vi "Three Button Dialog CORE-WithTimeout.vi"(0 "message":string, 1 "Window Title (\"\")":string, 3 "Justify Message (Left)":enum16{"Left", "Center", "Right"}(ring), 7 "Timeout(s)":i32=-1, 11 "error in (no error)":errorcluster, 12 "Keyboard Shortcuts (Left is <Enter>)":T1={"Left Button Key Shortcut"={"Control"=FALSE, "Shift"=FALSE, "Key"="<Enter>"}, "Center Button Key Shortcut"={"Control"=FALSE, "Shift"=FALSE, "Key"=""}, "Right Button Key Shortcut"={"Control"=FALSE, "Shift"=FALSE, "Key"=""}}, 13 "Enable(t)":bool=TRUE, 14 "Allow user to close window? (TRUE)":bool=TRUE) -> (2 "OK(?)":bool, 4 "Which Button?":T2(ring)=enum."Center Button", 15 "error out":errorcluster)   [LabVIEW 2018]
doc: "Displays text in a dialog with three buttons. The output enum indicates which of the three buttons the user chose, or it indicates that the user closed the dialog without making any choice."
uses:
  <vilib>/Utility/miscctls.llb/LVRectTypeDef.ctl
panel:
  in  "OK":string="OK"
  out "C-Message":string
  in  "Right Button":bool
  in  "Center Button":bool
  in  "Left Button":bool
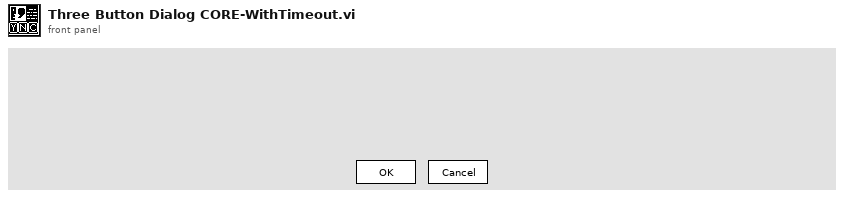
[diagram p1: front panel]
types:
  T1 = cluster{"Left Button Key Shortcut":cluster{"Control":bool, "Shift":bool, "Key":string}, "Center Button Key Shortcut":cluster{"Control":bool, "Shift":bool, "Key":string}, "Right Button Key Shortcut":cluster{"Control":bool, "Shift":bool, "Key":string}}
  T2 = enum16{"Left Button", "Center Button", "Right Button", "Window Close"}
  T3 = cluster{"left":i16, "top":i16, "right":i16, "bottom":i16}
  T4 = cluster{"Control":bool, "Shift":bool, "Key":string}
  T5 = cluster{bool, "Control":bool, "Shift":bool, "Key":string}
  T6 = typedef "LVRectTypeDef.ctl" = cluster{"Left":i16, "Top":i16, "Right":i16, "Bottom":i16}
  T7 = typedef "LVBoundsTypeDef.ctl" = cluster{"Width":u32, "Height":u32}
  T8 = typedef "LVPointTypeDef.ctl" = cluster{"Horizontal":i16, "Vertical":i16}
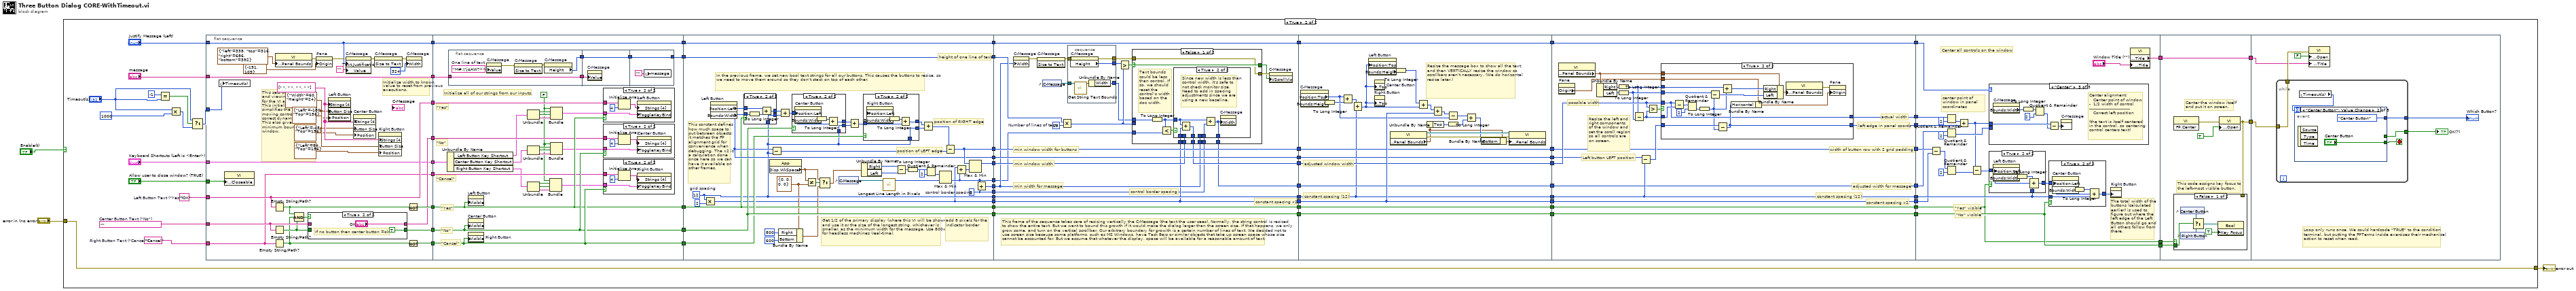
[diagram p0: block diagram]
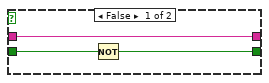
[diagram p3: hidden frame]
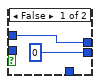
[diagram p7: hidden frame]
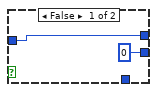
[diagram p8: hidden frame]
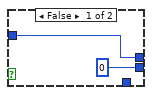
[diagram p9: hidden frame]
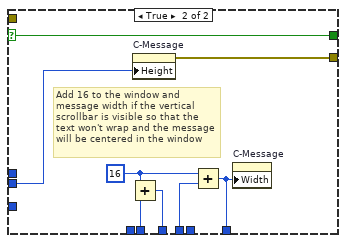
[diagram p11: hidden frame]
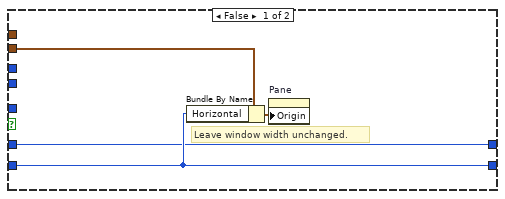
[diagram p12: hidden frame]
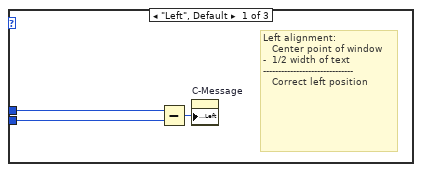
[diagram p13: hidden frame]
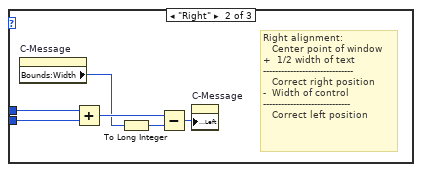
[diagram p14: hidden frame]
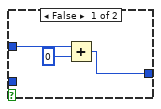
[diagram p15: hidden frame]
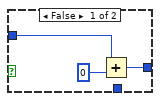
[diagram p16: hidden frame]
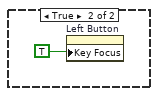
[diagram p17: hidden frame]
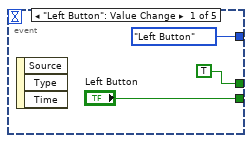
[diagram p18: hidden frame]
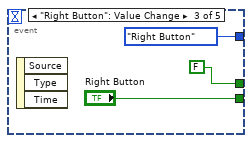
[diagram p19: hidden frame]
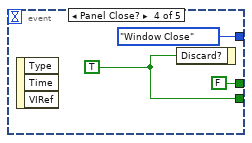
[diagram p20: hidden frame]
diagram:
  n1 = case shown="True" "Enable(t)" {
    tunnel: "error in (no error)" -> [_ w9]
    tunnel: [_ w9] -> w1
    frame False {
    }
    frame True {
      w15 = "Cancel"  # Right Button Text ("Cancel")
      w16 = ""  # Center Button Text ("No")
      w17 = "OK"  # Left Button Text ("Yes")
      n2 = Equal?(x=-1, y="Timeout(s)") -> (x = y?=w5:bool)
      n3 = Multiply(x="Timeout(s)", y=1000) -> (x*y=w8:i32)
      n4 = Select(t="Timeout(s)", s=w5, f=w8) -> (s? t:f=w4:i32)
      n5 = flat-sequence {
        tunnel: [w94] -> w75
        tunnel: [w96] -> w74
        tunnel: [w95] -> w73
        tunnel: [w90] -> w72
        tunnel: [w91] -> w71
        tunnel: [w88] -> w70
        tunnel: [w87] -> w69
        tunnel: w17 -> [w90]
        tunnel: w16 -> [w89]
        tunnel: w15 -> [w88]
        tunnel: "Justify Message (Left)" -> [w87]
        tunnel: "Keyboard Shortcuts (Left is <Enter>)" -> [w84]
        tunnel: [w84] -> w68
        tunnel: "message" -> [w83]
        tunnel: [w83] -> w67
        tunnel: "Allow user to close window? (TRUE)" -> [w82]
        tunnel: w4 -> [w76]
        tunnel: w75 -> [w138]
        tunnel: [w138] -> w66
        tunnel: w74 -> [w137]
        tunnel: [w137] -> w65
        tunnel: w73 -> [w136]
        tunnel: [w136] -> w64
        tunnel: w72 -> [w135]
        tunnel: w71 -> [w134]
        tunnel: w70 -> [w133]
        tunnel: w69 -> [w132]
        tunnel: [w132] -> w63
        tunnel: [w128] -> w62
        tunnel: w68 -> [w131]
        tunnel: w67 -> [w127]
        tunnel: [w199] -> w61
        tunnel: [w196] -> w60
        tunnel: [w195] -> w59
        tunnel: [w178] -> w58
        tunnel: [w160] -> w57
        tunnel: w66 -> [w188]
        tunnel: w65 -> [w190]
        tunnel: [w190] -> w56
        tunnel: w64 -> [w186]
        tunnel: [w186] -> w55
        tunnel: [w171] -> w54
        tunnel: w63 -> [w181]
        tunnel: [w181] -> w53
        tunnel: w62 -> [w180]
        tunnel: [w180] -> w52
        tunnel: [w169] -> w51
        tunnel: [w168] -> w50
        tunnel: w61 -> [w234]
        tunnel: [w233] -> w49
        tunnel: w60 -> [w240]
        tunnel: [w240] -> w48
        tunnel: w59 -> [w239]
        tunnel: [w239] -> w47
        tunnel: w58 -> [w238]
        tunnel: [w238] -> w46
        tunnel: w57 -> [w227]
        tunnel: [w227] -> w45
        tunnel: w56 -> [w237]
        tunnel: [w237] -> w44
        tunnel: w55 -> [w236]
        tunnel: [w236] -> w43
        tunnel: w54 -> [w228]
        tunnel: [w232] -> w42
        tunnel: w53 -> [w235]
        tunnel: [w235] -> w41
        tunnel: w52 -> [w230]
        tunnel: w51 -> [w226]
        tunnel: w50 -> [w225]
        tunnel: w49 -> [w289]
        tunnel: [w289] -> w40
        tunnel: w48 -> [w288]
        tunnel: [w288] -> w39
        tunnel: w47 -> [w287]
        tunnel: [w287] -> w38
        tunnel: w46 -> [w280]
        tunnel: [w280] -> w37
        tunnel: w45 -> [w297]
        tunnel: [w297] -> w36
        tunnel: w44 -> [w286]
        tunnel: [w286] -> w35
        tunnel: w43 -> [w285]
        tunnel: [w285] -> w34
        tunnel: w42 -> [w284]
        tunnel: [w284] -> w33
        tunnel: w41 -> [w283]
        tunnel: [w283] -> w32
        tunnel: w40 -> [w324]
        tunnel: [w319] -> w31
        tunnel: w39 -> [w312]
        tunnel: [w312] -> w30
        tunnel: w38 -> [w318]
        tunnel: w37 -> [w317]
        tunnel: [w317] -> w29
        tunnel: w36 -> [w311]
        tunnel: [w311] -> w28
        tunnel: [w315] -> w27
        tunnel: w35 -> [w310]
        tunnel: [w310] -> w26
        tunnel: w34 -> [w309]
        tunnel: [w309] -> w25
        tunnel: w33 -> [w306]
        tunnel: [w306] -> w24
        tunnel: w32 -> [w308]
        tunnel: [w308] -> w23
        tunnel: [w349] -> w22
        tunnel: w31 -> [w368]
        tunnel: w30 -> [w361]
        tunnel: w29 -> [w365]
        tunnel: w28 -> [w360]
        tunnel: w27 -> [w367]
        tunnel: w26 -> [w348]
        tunnel: w25 -> [w347]
        tunnel: w24 -> [w353]
        tunnel: w23 -> [w354]
        tunnel: [w348] -> w21
        tunnel: [w347] -> w20
        tunnel: w22 -> [w404]
        tunnel: w21 -> [w400]
        tunnel: w20 -> [w401]
        tunnel: [w402] -> w19
        tunnel: [w404] -> w18
        tunnel: w19 -> [w412]
        tunnel: w18 -> [w413]
        frame #0 {
          w104 = string[] [" ", " ", " ", " "] ("Strings [4]")
          w103 = cluster{"Width":u32, "Height":u32} {"Width"=60, "Height"=24} ("Button Size")
          # "Initialize width to known value to reset from previous executions."
          # "This sets up initial sizes and viewing rectangles\nfor the VI and its controls. This initialization\nsimplifies the task of moving controls to their\ncorrect dynamic locations. This also gives us our\nminimum bounds for the window."
          n6 = local write "Timeout(s)"(w76) -> ()
          n7 = property class="VI"("Front Panel Window:Closeable"=w82) -> ()  [unwired: 2 in, 2 out]
          n8 = Empty String/Path?(string/path=w90) -> (empty?=w98:bool)
          n9 = Empty String/Path?(string/path=w89) -> (empty?=w86:bool)
          n10 = Empty String/Path?(string/path=w88) -> (empty?=w85:bool)
          n11 = property class="VI"("Front Panel Window:Panel Bounds"=T3 {"left"=338, "top"=316, "right"=686, "bottom"=392} ("Front Panel.PanelBounds")) -> (error out=w81:errorcluster)  [unwired: 2 in, 1 out]
          n12 = Compound Arithmetic op=AND(w98, w85, w86) -> (w97:bool)
          n13 = case shown="True" w97 {
            tunnel: w86 -> [w107 _]
            tunnel: [w106 TRUE] -> w96
            tunnel: w89 -> [w105 _]
            tunnel: [w105 "OK"] -> w91
            frame False {
              n14 = Not(x=w107) -> (.not. x?=w106:bool)
            }
            frame True {
              # "If no button then center button =ok"
            }
          }
          n15 = property on="Pane" class="Pane"(error in=w81, "Origin"=cluster{"Horizontal":i16, "Vertical":i16} {"Horizontal"=-191, "Vertical"=109} ("Front Panel.Origin")) -> (error out=w80:errorcluster)  [unwired: 1 in, 1 out]
          n16 = property on="Left Button" class="Bool"("Strings [4]"=w104, "Button Size"=w103, "Position"=cluster{"Left":i32, "Top":i32} {"Left"=-180, "Top"=156}) -> ()  [unwired: 2 in, 2 out]
          n17 = property on="C-Message" class="Str"(error in=w80, "Text.Justification"=w87, "Value"="") -> (error out=w99:errorcluster)  [unwired: 1 in, 1 out]
          n18 = property on="Center Button" class="Bool"("Strings [4]"=w104, "Button Size"=w103, "Position"=cluster{"Left":i32, "Top":i32} {"Left"=-48, "Top"=156}) -> ()  [unwired: 2 in, 2 out]
          n19 = invoke on="C-Message" class="Str" method="Size to Text"(error in=w99) -> (error out=w78:errorcluster)  [unwired: 2 in, 2 out]
          n20 = property on="Right Button" class="Bool"("Strings [4]"=w104, "Button Size"=w103, "Position"=cluster{"Left":i32, "Top":i32} {"Left"=84, "Top"=156}) -> ()  [unwired: 2 in, 2 out]
          n21 = property on="C-Message" class="Str"(error in=w78, "Width"=u32 324 ("Size:Width")) -> ()  [unwired: 1 in, 2 out]
          n22 = Not(x=w98) -> (.not. x?=w95:bool)
          n23 = Not(x=w85) -> (.not. x?=w94:bool)
        }
        frame #1 {
          w112 = FALSE
          # "\"Cancel\""
          # "\"No\""
          # "\"Yes\""
          # "\"Cancel\""
          # "\"No\""
          # "\"Yes\""
          # "Initialize all of our strings from our inputs."
          n24 = Unbundle By Name(w131) -> ("Left Button Key Shortcut"=w125:T4, "Center Button Key Shortcut"=w117:T4, "Right Button Key Shortcut"=w111:T4)
          n25 = flat-sequence {
            tunnel: [w140] -> w130
            tunnel: w127 -> [w139]
            tunnel: [w139] -> w126
            tunnel: w130 -> [w145]
            tunnel: [w145] -> w129
            tunnel: w126 -> [w144]
            tunnel: w129 -> [w146]
            tunnel: [w146] -> w128
            frame #0 {
              w143 = "M#,\"jqAW?><"  # One line of text
              n26 = property on="C-Message" class="Str"("Value"=w143) -> (error out=w141:errorcluster)  [unwired: 2 in, 1 out]
              n27 = invoke on="C-Message" class="Str" method="Size to Text"(error in=w141) -> (error out=w142:errorcluster)  [unwired: 2 in, 2 out]
              n28 = property on="C-Message" class="Str"(error in=w142) -> ("Height"=w140:u32)  [unwired: 1 in, 2 out]
            }
            frame #1 {
              n29 = property on="C-Message" class="Str"("Value"=w144) -> ()  [unwired: 2 in, 2 out]
            }
            frame #2 {
              n30 = local write "message"("") -> ()
            }
          }
          n31 = property on="Left Button" class="Bool"("Visible"=w136) -> ()  [unwired: 2 in, 2 out]
          n32 = property on="Center Button" class="Bool"("Visible"=w137) -> ()  [unwired: 2 in, 2 out]
          n33 = property on="Right Button" class="Bool"("Visible"=w138) -> ()  [unwired: 2 in, 2 out]
          n34 = Unbundle(w125) -> ("Control"=w124:bool, "Shift"=w123:bool, "Key"=w122:string)
          n35 = Unbundle(w117) -> ("Control"=w120:bool, "Shift"=w119:bool, "Key"=w118:string)
          n36 = Unbundle(w111) -> ("Control"=w115:bool, "Shift"=w114:bool, "Key"=w113:string)
          n37 = Bundle(w112, "Control"=w115, "Shift"=w114, "Key"=w113) -> (w110:T5)  [unwired: 1 in]
          n38 = Bundle(w112, "Control"=w124, "Shift"=w123, "Key"=w122) -> (w121:T5)  [unwired: 1 in]
          n39 = Bundle(w112, "Control"=w120, "Shift"=w119, "Key"=w118) -> (w116:T5)  [unwired: 1 in]
          n40 = case shown="True" w136 {
            tunnel: w135 -> [_ w157]
            tunnel: w121 -> [_ w156]
            frame False {
            }
            frame True {
              n41 = Initialize Array(w157, 4 ("dimension size")) -> (w159:string[])
              n42 = property on="Left Button" class="Bool"("Strings [4]"=w159, "ToggleKeyBind"=w156) -> ()  [unwired: 2 in, 2 out]
            }
          }
          n43 = case shown="True" w137 {
            tunnel: w116 -> [_ w153]
            tunnel: w134 -> [_ w152]
            frame False {
            }
            frame True {
              n44 = Initialize Array(w152, 4 ("dimension size")) -> (w155:string[])
              n45 = property on="Center Button" class="Bool"("Strings [4]"=w155, "ToggleKeyBind"=w153) -> ()  [unwired: 2 in, 2 out]
            }
          }
          n46 = case shown="True" w138 {
            tunnel: w110 -> [_ w149]
            tunnel: w133 -> [_ w148]
            frame False {
            }
            frame True {
              n47 = Initialize Array(w148, 4 ("dimension size")) -> (w151:string[])
              n48 = property on="Right Button" class="Bool"("Strings [4]"=w151, "ToggleKeyBind"=w149) -> ()  [unwired: 2 in, 2 out]
            }
          }
        }
        frame #2 {
          w165 = T6 {"Left"=0, "Top"=0, "Right"=0, "Bottom"=0} ("Display:Primary Workspace")
          w169 = 8  # control border spacing
          w178 = 12  # grid spacing
          # "position of RIGHT edge"
          # "height of one line of text"
          # "add 8 pixels for the indicator border"
          # "Get 1/2 of the primary display (where this VI will be shown) and use it or the size of the longest string, whichever is smaller, as the minimum width for the message. Use 800x600 for headless machines (real-time)."
          # "This constant defines how much space to put between objects; it matches the FP alignment grid for convenience when debugging. The x2 is a calculation done once here so we can have it available on other frames."
          # "In the previous frame, we set new bool text strings for all our buttons. This causes the buttons to resize, so we need to move them around so they don't stack on top of each other."
          # "position of LEFT edge"
          n49 = Multiply(x=w178, y=2) -> (x*y=w160:i32)
          n50 = property on="Left Button" class="Bool"() -> ("Position:Left"=w195:i32, "Bounds:Width"=w192:u32)  [unwired: 2 in, 2 out]
          n51 = case shown="True" w186 {
            tunnel: w195 -> [w202 w207]
            tunnel: w192 -> [_ w206]
            tunnel: [w202 w205] -> w187
            tunnel: w178 -> [_ w203]
            tunnel: [0 w203] -> w185
            frame False {
            }
            frame True {
              n52 = To Long Integer(number=w206) -> (32bit integer=w204:i32)
              n53 = Add(x=w207, y=w204) -> (x+y=w205:i32)
            }
          }
          n54 = property class="App"() -> ("Disp.WkSpace"=w166:T6)  [unwired: 2 in, 2 out]
          n55 = Subtract(x=w195, y=w178) -> (x-y=w197:i32)
          n56 = Bundle By Name(cluster=w165, "Right"=i16 800, "Bottom"=i16 600) -> (w162:T6)
          n57 = Add(x=w187, y=w185) -> (x+y=w193:i32)
          n58 = case shown="True" w190 {
            tunnel: w193 -> [w216 w221]
            tunnel: [w216 w220] -> w191
            tunnel: [0 w217] -> w184
            tunnel: w178 -> [_ w217]
            frame False {
            }
            frame True {
              n59 = property on="Center Button" class="Bool"("Position:Left"=w221) -> ("Bounds:Width"=w219:u32)  [unwired: 2 in, 2 out]
              n60 = To Long Integer(number=w219) -> (32bit integer=w218:i32)
              n61 = Add(x=w218, y=w221) -> (x+y=w220:i32)
            }
          }
          n62 = Not Equal?(x=w166, y=w165) -> (x != y?=w167:bool)
          n63 = Select(t=w166, s=w167, f=w162) -> (s? t:f=w161:T6)
          n64 = control-ref of="C-Message"() -> (w182:refnum<vi>)
          n65 = Add(x=w191, y=w184) -> (x+y=w194:i32)
          n66 = Unbundle By Name(w161) -> ("Right"=w174:i16, "Left"=w173:i16)
          n67 = case shown="True" w188 {
            tunnel: w194 -> [w209 w214]
            tunnel: [w209 w210] -> w189
            tunnel: [0 w211] -> w183
            tunnel: w178 -> [_ w211]
            frame False {
            }
            frame True {
              n68 = property on="Right Button" class="Bool"("Position:Left"=w214) -> ("Bounds:Width"=w213:u32)  [unwired: 2 in, 2 out]
              n69 = To Long Integer(number=w213) -> (32bit integer=w212:i32)
              n70 = Add(x=w212, y=w214) -> (x+y=w210:i32)
            }
          }
          n71 = call <vilib>:"Longest Line Length in Pixels.vi"("String"=w182) -> ("longest line length"=w175:i32)  [unwired: 9 in]
          n72 = Subtract(x=w174, y=w173) -> (x-y=w177:i16)
          n73 = To Long Integer(number=w177) -> (32bit integer=w172:i32)
          n74 = Add(x=w189, y=w183) -> (x+y=w198:i32)
          n75 = Quotient & Remainder(x=w172, y=2) -> (floor(x/y)=w170:i32)  [unwired: 1 out]
          n76 = Max & Min(x=w170, y=w175) -> (min(x,y)=w168:i32)  [unwired: 1 out]
          n77 = Subtract(x=w198, y=w197) -> (x-y=w196:i32)
          n78 = Add(x=w160, y=w168) -> (x+y=w200:i32)
          n79 = Max & Min(x=w196, y=w200) -> (max(x,y)=w199:i32)  [unwired: 1 out]
          n80 = Add(x=w168, y=w169) -> (x+y=w171:i32)
        }
        frame #3 {
          w242 = u32 25  # Number of lines of text
          # "control border spacing"
          # "constant spacing x2"
          # "min window width for buttons"
          # "min window width"
          # "min width for message"
          # "This frame of the sequence takes care of resizing vertically the C-Message (the text the user sees). Normally, the string control is resized to show the entire text. But we want to bound this growth if it would make the dialog larger than the screen size. If that happens, we only grow some, and turn on the vertical scrollbar. Our arbitrary boundary for growith is a certain number of lines of text. We decided not to use screen size because some platforms, such as MS Windows, have Task Bars or similar objects that take up screen space whose size cannot be accounted for. But we assume that whatever the display, space will be available for a reasonable amount of text."
          n81 = property on="C-Message" class="Str"("Width"=w228) -> (error out=w231:errorcluster)  [unwired: 2 in, 1 out]
          n82 = invoke on="C-Message" class="Str" method="Size to Text"(error in=w231) -> (error out=w246:errorcluster)  [unwired: 2 in, 2 out]
          n83 = control-ref of="C-Message"() -> (w223:refnum<vi>)
          n84 = Multiply(x=w230, y=w242) -> (x*y=w241:u32)
          n85 = stacked-sequence {
            tunnel: w246 -> [w252]
            tunnel: [w251] -> w229
            tunnel: [w250] -> w224
            tunnel: w223 -> [w249]
            tunnel: [w247] -> w222
            frame #0 {
              n86 = property on="C-Message" class="Str"(error in=w252) -> (error out=w250:errorcluster, "Height"=w251:u32)  [unwired: 1 in, 1 out]
              n87 = call <vilib>:"Get String Text Bounds.vi"("String"=w249) -> ("Text bounds"=w248:T7)  [unwired: 10 in]
              n88 = Unbundle By Name(w248) -> ("Width"=w247:u32)
            }
          }
          n89 = Greater?(x=w229, y=w241) -> (0:w245:bool)
          n90 = case shown="False" w245 {
            selector: w245 -> [w264 w278]
            tunnel: [w263 w279] -> w244
            tunnel: [w264 w278] -> w243
            tunnel: w224 -> [w263 _]
            tunnel: w241 -> [_ w277]
            tunnel: [w257 w275] -> w233
            tunnel: w234 -> [w259 w276]
            tunnel: [w256 w272] -> w232
            tunnel: w228 -> [w258 w274]
            tunnel: w222 -> [w261 _]
            tunnel: w225 -> [w260 _]
            tunnel: w227 -> [w255 _]
            tunnel: w226 -> [w254 _]
            frame False {
              # "Text bounds could be less than control. If so, we should reset the control's width based on the doc width."
              n91 = To Long Integer(number=w261) -> (32bit integer=w253:i32)
              n92 = Less?(x=w253, y=w260) -> (x < y?=w262:bool)
              n93 = case shown="True" w262 {
                tunnel: w253 -> [_ w270]
                tunnel: w259 -> [w266 _]
                tunnel: w258 -> [w265 _]
                tunnel: [w266 w269] -> w257
                tunnel: [w265 w268] -> w256
                tunnel: w255 -> [_ w271]
                tunnel: w254 -> [_ w267]
                frame False {
                }
                frame True {
                  # "Since new width is less than control width, it's safe to not check monitor size. \nNeed to add in spacing adjustments since we are using a new baseline."
                  n94 = Add(x=w270, y=w271) -> (x+y=w269:i32)
                  n95 = Add(x=w270, y=w267) -> (x+y=w268:i32)
                  n96 = property on="C-Message" class="Str"("Width"=w268) -> ()  [unwired: 2 in, 2 out]
                }
              }
            }
            frame True {
              w273 = 16 ("x")
              # "Add 16 to the window and message width if the vertical scrollbar is visible so that the text won't wrap and the message will be centered in the window"
              n97 = Add(x=w273, y=w276) -> (x+y=w275:i32)
              n98 = property on="C-Message" class="Str"("Height"=w277) -> (error out=w279:errorcluster)  [unwired: 2 in, 1 out]
              n99 = Add(x=w273, y=w274) -> (x+y=w272:i32)
              n100 = property on="C-Message" class="Str"("Width"=w272) -> ()  [unwired: 2 in, 2 out]
            }
          }
          n101 = property on="C-Message" class="Str"(error in=w244, "VScrollVis"=w243) -> ()  [unwired: 1 in, 2 out]
        }
        frame #4 {
          # "adjusted window width"
          # "constant spacing (12)"
          # "Resize the message box to show all the text, and then VERTICALLY resize the window so scrollbars aren't necessary. (We do horizontal resize later.)"
          n102 = property on="C-Message" class="Str"() -> ("Position:Top"=w291:i32, "Bounds:Height"=w290:u32)  [unwired: 2 in, 2 out]
          n103 = To Long Integer(number=w290) -> (32bit integer=w296:i32)
          n104 = Add(x=w291, y=w296) -> (x+y=w281:i32)
          n105 = Add(x=w281, y=w280) -> (x+y=w282:i32)
          n106 = property on="Left Button" class="Bool"("Position:Top"=w282) -> ("Bounds:Height"=w293:u32)  [unwired: 2 in, 2 out]
          n107 = property on="Center Button" class="Bool"("Position:Top"=w282) -> ()  [unwired: 2 in, 2 out]
          n108 = property on="Right Button" class="Bool"("Position:Top"=w282) -> ()  [unwired: 2 in, 2 out]
          n109 = property class="VI"() -> (reference out=w303:refnum<vi>, error out=w304:errorcluster, "Front Panel Window:Panel Bounds"=w294:T6)  [unwired: 2 in]
          n110 = To Long Integer(number=w293) -> (32bit integer=w292:i32)
          n111 = Add(x=w292, y=w282) -> (x+y=w298:i32)
          n112 = Unbundle By Name(w294) -> ("Top"=w301:i16)
          n113 = Add(x=w298, y=w297) -> (x+y=w299:i32)
          n114 = Subtract(x=w299, y=w291) -> (x-y=w302:i32)
          n115 = To Long Integer(number=w301) -> (32bit integer=w295:i32)
          n116 = Add(x=w302, y=w295) -> (x+y=w300:i32)
          n117 = Bundle By Name(cluster=w294, "Bottom"=w300) -> (w305:T6)
          n118 = property class="VI"(reference=w303, error in=w304, "Front Panel Window:Panel Bounds"=w305) -> ()  [unwired: 2 out]
        }
        frame #5 {
          # "adjusted width for message"
          # "constant spacing x2"
          # "constant spacing (12)"
          # "Left button LEFT position"
          # "left edge in panel coords"
          # "width of button row with 2 grid padding"
          # "Resize the left and\nright components\nof the window and\nset the scroll region\nso all controls are \non screen."
          # "actual width"
          # "possible width"
          n119 = property class="VI"() -> ("Front Panel Window:Panel Bounds"=w321:T6)  [unwired: 2 in, 2 out]
          n120 = property on="Pane" class="Pane"() -> ("Origin"=w307:T8)  [unwired: 2 in, 2 out]
          n121 = Unbundle By Name(w321) -> ("Right"=w323:i16, "Left"=w322:i16)
          n122 = To Long Integer(number=w323) -> (32bit integer=w313:i32)
          n123 = To Long Integer(number=w322) -> (32bit integer=w314:i32)
          n124 = Subtract(x=w313, y=w314) -> (x-y=w325:i32)
          n125 = Subtract(x=w318, y=w317) -> (x-y=w316:i32)
          n126 = Greater?(x=w324, y=w325) -> (0:w320:bool)
          n127 = case shown="True" w320 {
            tunnel: w325 -> [w327 w346]
            tunnel: w324 -> [_ w333]
            tunnel: w313 -> [_ w341]
            tunnel: w314 -> [_ w342]
            tunnel: w321 -> [_ w343]
            tunnel: [w329 w335] -> w319
            tunnel: w307 -> [w328 w336]
            tunnel: w316 -> [w329 w334]
            tunnel: [w327 w333] -> w315
            frame False {
              # "Leave window width unchanged."
              n128 = Bundle By Name(cluster=w328, "Horizontal"=w329) -> (w326:T8)
              n129 = property on="Pane" class="Pane"("Origin"=w326) -> ()  [unwired: 2 in, 2 out]
            }
            frame True {
              n130 = Subtract(x=w333, y=w346) -> (x-y=w345:i32)
              n131 = Quotient & Remainder(x=w345, y=2) -> (floor(x/y)=w338:i32)  [unwired: 1 out]
              n132 = To Long Integer(number=w338) -> (32bit integer=w332:i32)
              n133 = Subtract(x=w342, y=w332) -> (x-y=w339:i32)
              n134 = Subtract(x=w334, y=w332) -> (x-y=w335:i32)
              n135 = Add(x=w341, y=w332) -> (x+y=w340:i32)
              n136 = Bundle By Name(cluster=w336, "Horizontal"=w335) -> (w330:T8)
              n137 = Bundle By Name(cluster=w343, "Right"=w340, "Left"=w339) -> (w337:T6)
              n138 = property class="VI"("Front Panel Window:Panel Bounds"=w337) -> (error out=w331:errorcluster)  [unwired: 2 in, 1 out]
              n139 = property on="Pane" class="Pane"(error in=w331, "Origin"=w330) -> ()  [unwired: 1 in, 2 out]
            }
          }
        }
        frame #6 {
          # "\"No\" visible"
          # "\"Yes\" visible"
          # "The total width of the buttons (calculated earlier) is used to figure out where the left edge of the Left Button should go and all others follow from there."
          # "center point of window in panel coordinates"
          # "Center all controls on the window"
          n140 = Subtract(x=w361, y=w360) -> (x-y=w362:i32)
          n141 = Quotient & Remainder(x=w367, y=2) -> (floor(x/y)=w364:i32)  [unwired: 1 out]
          n142 = Quotient & Remainder(x=w353, y=2) -> (floor(x/y)=w352:i32)  [unwired: 1 out]
          n143 = Quotient & Remainder(x=w362, y=2) -> (floor(x/y)=w359:i32)  [unwired: 1 out]
          n144 = Add(x=w364, y=w368) -> (x+y=w351:i32)
          n145 = Subtract(x=w351, y=w359) -> (x-y=w358:i32)
          n146 = case shown="\"Center\"" w354 {
            tunnel: w351 -> [w371 w377 w379]
            tunnel: w352 -> [w369 w376 _]
            frame "Left", Default {
              # "Left alignment:\n   Center point of window\n-  1/2 width of text\n------------------------------\n   Correct left position"
              n147 = Subtract(x=w371, y=w369) -> (x-y=w370:i32)
              n148 = property on="C-Message" class="Str"("Position:Left"=w370) -> ()  [unwired: 2 in, 2 out]
            }
            frame "Right" {
              # "Right alignment:\n   Center point of window\n+  1/2 width of text\n------------------------------\n   Correct right position\n-  Width of control\n-----------------------------\n   Correct left position"
              n149 = property on="C-Message" class="Str"() -> ("Bounds:Width"=w373:u32)  [unwired: 2 in, 2 out]
              n150 = Add(x=w377, y=w376) -> (x+y=w375:i32)
              n151 = To Long Integer(number=w373) -> (32bit integer=w372:i32)
              n152 = Subtract(x=w375, y=w372) -> (x-y=w374:i32)
              n153 = property on="C-Message" class="Str"("Position:Left"=w374) -> ()  [unwired: 2 in, 2 out]
            }
            frame "Center" {
              # "Center alignment:\n   Center point of window\n-  1/2 width of control\n------------------------------\n   Correct left position\n\n(the text is itself centered in the control, so centering control centers text)"
              n154 = property on="C-Message" class="Str"() -> ("Bounds:Width"=w382:u32)  [unwired: 2 in, 2 out]
              n155 = To Long Integer(number=w382) -> (32bit integer=w380:i32)
              n156 = Quotient & Remainder(x=w380, y=2) -> (floor(x/y)=w378:i32)  [unwired: 1 out]
              n157 = Subtract(x=w379, y=w378) -> (x-y=w381:i32)
              n158 = property on="C-Message" class="Str"("Position:Left"=w381) -> ()  [unwired: 2 in, 2 out]
            }
          }
          n159 = case shown="True" w347 {
            tunnel: w365 -> [_ w399]
            tunnel: w358 -> [w394 w398]
            tunnel: [w393 w396] -> w357
            frame False {
              n160 = Add(x=w394, y=0) -> (x+y=w393:i32)
            }
            frame True {
              n161 = property on="Left Button" class="Bool"("Position:Left"=w398) -> ("Bounds:Width"=w397:u32)  [unwired: 2 in, 2 out]
              n162 = To Long Integer(number=w397) -> (32bit integer=w395:i32)
              n163 = Compound Arithmetic op=ADD(w395, w398, w399) -> (w396:i32)
            }
          }
          n164 = case shown="True" w348 {
            tunnel: w365 -> [_ w391]
            tunnel: w357 -> [w386 w389]
            tunnel: [w385 w388] -> w356
            frame False {
              n165 = Add(x=w386, y=0) -> (x+y=w385:i32)
            }
            frame True {
              n166 = property on="Center Button" class="Bool"("Position:Left"=w389) -> ("Bounds:Width"=w390:u32)  [unwired: 2 in, 2 out]
              n167 = To Long Integer(number=w390) -> (32bit integer=w387:i32)
              n168 = Compound Arithmetic op=ADD(w387, w389, w391) -> (w388:i32)
            }
          }
          n169 = property on="Right Button" class="Bool"("Position:Left"=w356) -> ()  [unwired: 2 in, 2 out]
          n170 = property class="VI"("Front Panel Window:Title"="Window Title (\"\")") -> ("Front Panel Window:Title"=w349:string)  [unwired: 2 in, 2 out]
        }
        frame #7 {
          # "This code assigns key focus to\nthe left-most visible button."
          # "Center the window itself and put it on screen."
          n171 = invoke class="VI" method="FP.Center"() -> (error out=w403:errorcluster)  [unwired: 3 in, 2 out]
          n172 = property class="VI"(error in=w403, "Front Panel Window:Open"=TRUE) -> (error out=w402:errorcluster)  [unwired: 1 in, 1 out]
          n173 = case shown="False" w401 {
            tunnel: w402 -> [_ _]
            tunnel: w400 -> [w410 _]
            frame False {
              n174 = control-ref of="Center Button"() -> (w409:refnum<vi>)
              n175 = control-ref of="Right Button"() -> (w408:refnum<vi>)
              n176 = Select(t=w409, s=w410, f=w408) -> (s? t:f=w407:refnum<vi>)
              n177 = property class="Bool"(reference=w407, "Key Focus"=TRUE) -> ()  [unwired: 1 in, 2 out]
            }
            frame True {
              n178 = property on="Left Button" class="Bool"("Key Focus"=TRUE) -> ()  [unwired: 2 in, 2 out]
            }
          }
        }
        frame #8 {
          # "Loop only runs once. We could hardcode \"TRUE\" to the condition terminal, but putting the FPTerms inside exercises their mechanical action to reset when read."
          n179 = while {
            tunnel: [w422] -> w415
            tunnel: [w421] -> w416
            tunnel: w412 -> [w421]
            tunnel: [w418] -> w417
            stop <- w420 stop-if-true
            n180 = local read "Timeout(s)"() -> (w419:i32)
            n181 = event shown="[1] \"Center Button\": Value Change" {
              selector: _ -> [_ _ _ _ _]
              dyn-events: _ -> [_ _ _ _ _]
              timeout: w419 -> [_ _ _ _ _]
              tunnel: ["Left Button" "Center Button" "Right Button" w432 w435] -> w420
              tunnel: [T2."Left Button" ("Which Button?") T2."Center Button" ("Which Button?") T2."Right Button" ("Which Button?") T2."Window Close" ("Which Button?") _] -> w422
              tunnel: [TRUE ("OK(?)") _ FALSE ("OK(?)") FALSE ("OK(?)") TRUE ("OK(?)")] -> w418
              event "Left Button": Value Change {
                n182 = event-data() -> ()  [unwired: 1 in, 3 out]
              }
              event "Center Button": Value Change {
                n183 = event-data() -> ()  [unwired: 1 in, 3 out]
              }
              event "Right Button": Value Change {
                n184 = event-data() -> ()  [unwired: 1 in, 3 out]
              }
              event Panel Close? {
                w432 = TRUE ("Discard?")
                n185 = event-data() -> ()  [unwired: 1 in, 3 out]
                n186 = event-data("Discard?"=w432) -> ()  [unwired: 1 in, 1 out]
              }
              event Timeout {
                n187 = event-data() -> ()  [unwired: 1 in, 3 out]
                n188 = for {
                  N: 3 -> [w439]
                  tunnel: [w437] -> w435
                  i -> [w440]
                  w442 = u32 1000 ("frequency (Hz)")
                  n189 = Increment(x=w440) -> (x+1=w438:i32)
                  n190 = call <vilib>:"Beep.vi"("use system alert? (T)"=FALSE, "duration (msec)"=w442, "frequency (Hz)"=w442) -> ()  [unwired: 9 in]
                  n191 = Equal?(x=w439, y=w438) -> (x = y?=w437:bool)
                }
              }
            }
          }
          "Which Button?" <- w415
          "OK(?)" <- w417
          n192 = property class="VI"(error in=w416, "Front Panel Window:Open"=FALSE, "Front Panel Window:Title"=w413) -> ()  [unwired: 1 in, 2 out]
        }
      }
    }
  }
  "error out" <- w1
